vi "Check Allowed Wheel Rotate.vi"(8 "error in (no error)":errorcluster, 10 "wheel index":i32, 11 "steering frame in":refnum<class "NI_Robotics_Steering Frame.lvclass">) -> (0 "error out":errorcluster, 2 "rotate allowed?":bool, 3 "steering frame out":refnum<class "NI_Robotics_Steering Frame.lvclass">)   [LabVIEW 2017, in "NI_Robotics_Configure Steering Frame.lvlib"]
uses:
  <vilib>/robotics/Dialog/Configure Steering Frame/NI_Robotics_Configure Steering Frame.lvlib
  <vilib>/robotics/Steering/Steering Frame/NI_Robotics_Steering Frame.lvclass
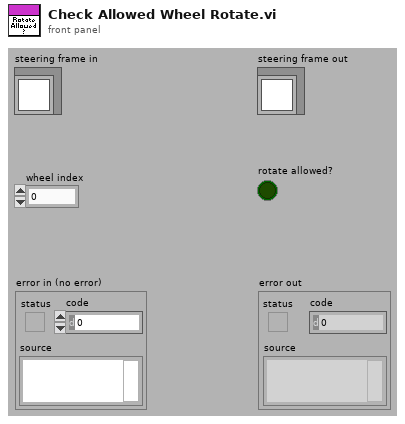
[diagram p1: front panel]
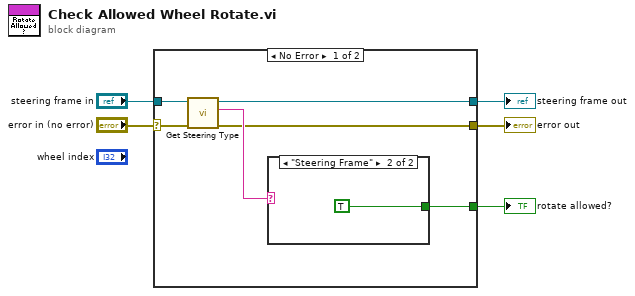
[diagram p0: block diagram]
diagram:
  n1 = case shown="No Error" "error in (no error)" {
    selector: "error in (no error)" -> [w10 w13]
    tunnel: "steering frame in" -> [w11 w14]
    tunnel: [w8 w14] -> w3
    tunnel: [w7 w13] -> w2
    tunnel: [w6 _] -> w1
    frame No Error {
      n2 = call-dynamic "Get Steering Type.vi"("error in (no error)"=w10, "steering frame in"=w11) -> ("error out"=w7:errorcluster, "steering type"=w9:string, "steering frame out"=w8:refnum<class "NI_Robotics_Steering Frame.lvclass">)  [unwired: 7 in]
      n3 = case shown="\"Steering Frame\"" w9 {
        tunnel: [_ TRUE] -> w6
        frame Default {
        }
        frame "Steering Frame" {
        }
      }
    }
    frame Error {
    }
  }
  "steering frame out" <- w3
  "error out" <- w2
  "rotate allowed?" <- w1
